vi "Read Target-FIFO 16ch.vi"(9 "ready for input":bool, 11 "channel number":u8) -> (4 "16xIQData":T1(array[cluster]) {"I" format="%.18g"; "Q" format="%.18g"}, 10 "Output Valid":bool)   [LabVIEW 2015, in "DDC_7976R_v1.lvlib"]
uses:
  DDC_7976R_v1.lvlib
types:
  T1 = cluster{"I":fxp<+/-,18,1>, "Q":fxp<+/-,18,1>, "overflow":bool}[]
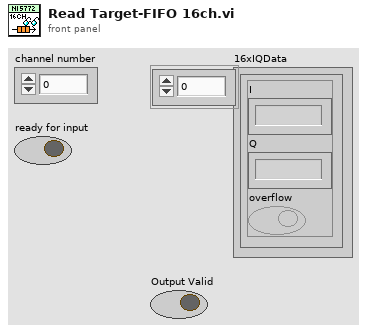
[diagram p1: front panel]
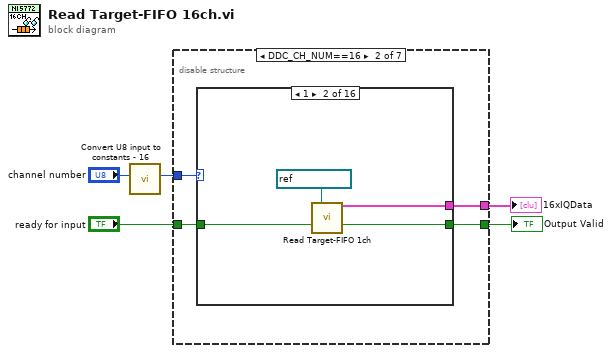
[diagram p0: block diagram]
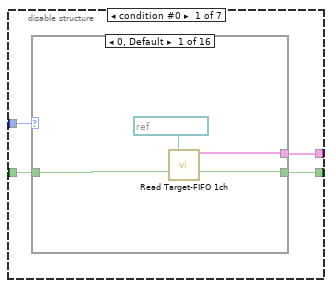
[diagram p2: hidden frame]
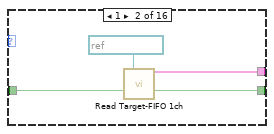
[diagram p3: hidden frame]
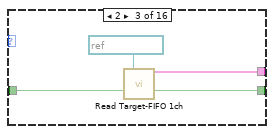
[diagram p4: hidden frame]
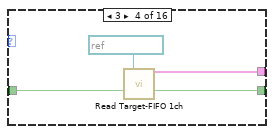
[diagram p5: hidden frame]
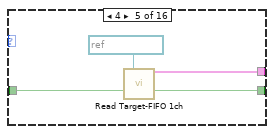
[diagram p6: hidden frame]
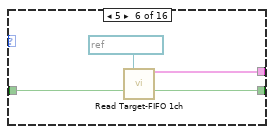
[diagram p7: hidden frame]
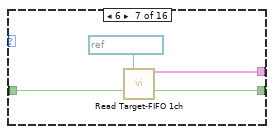
[diagram p8: hidden frame]
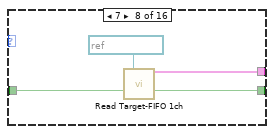
[diagram p9: hidden frame]
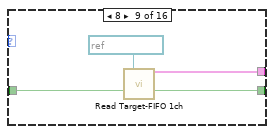
[diagram p10: hidden frame]
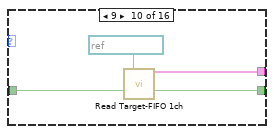
[diagram p11: hidden frame]
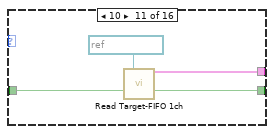
[diagram p12: hidden frame]
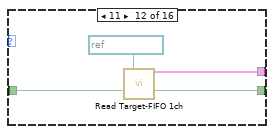
[diagram p13: hidden frame]
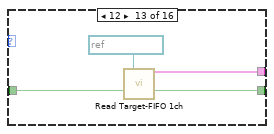
[diagram p14: hidden frame]
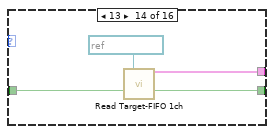
[diagram p15: hidden frame]
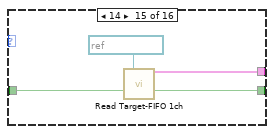
[diagram p16: hidden frame]
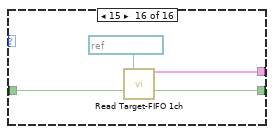
[diagram p17: hidden frame]
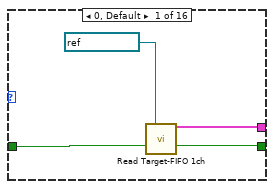
[diagram p18: hidden frame]
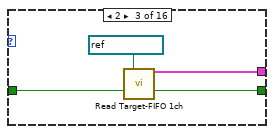
[diagram p19: hidden frame]
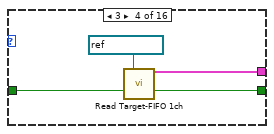
[diagram p20: hidden frame]
diagram:
  n1 = call "Convert U8 input to constants - 16.vi"("input U8"="channel number") -> ("output U8"=w1:u8)  [unwired: 10 in]
  n2 = disable-structure shown="DDC_CH_NUM==16" {
    disable-tunnel: [w9 w77 w145 w213 w281 w349 w415] -> w5
    disable-tunnel: [w8 w76 w144 w212 w280 w348 w416] -> w4
    disable-tunnel: "ready for input" -> [w7 w75 w143 w211 w279 w347 w414]
    disable-tunnel: w1 -> [w6 w74 w142 w210 w278 w346 _]
    frame condition #0 {
      n3 = case shown="0, Default" w6 {
        tunnel: w7 -> [w12 w16 w20 w24 w28 w32 w36 w40 w44 w48 w52 w56 w60 w64 w68 w72]
        tunnel: [w10 w15 w19 w23 w27 w31 w35 w39 w43 w47 w51 w55 w59 w63 w67 w71] -> w8
        tunnel: [w11 w14 w18 w22 w26 w30 w34 w38 w42 w46 w50 w54 w58 w62 w66 w70] -> w9
        frame 0, Default {
          n4 = call "Read Target-FIFO 1ch.vi"("FIFO In"=refnum<k21> "FIFO-000", "ready for input"=w12) -> ("16xIQData"=w10:T1, "Output Valid"=w11:bool)  [unwired: 12 in]
        }
        frame 1 {
          n5 = call "Read Target-FIFO 1ch.vi"("FIFO In"=refnum<k21> "FIFO-001", "ready for input"=w16) -> ("16xIQData"=w15:T1, "Output Valid"=w14:bool)  [unwired: 12 in]
        }
        frame 2 {
          n6 = call "Read Target-FIFO 1ch.vi"("FIFO In"=refnum<k21> "FIFO-002", "ready for input"=w20) -> ("16xIQData"=w19:T1, "Output Valid"=w18:bool)  [unwired: 12 in]
        }
        frame 3 {
          n7 = call "Read Target-FIFO 1ch.vi"("FIFO In"=refnum<k21> "FIFO-003", "ready for input"=w24) -> ("16xIQData"=w23:T1, "Output Valid"=w22:bool)  [unwired: 12 in]
        }
        frame 4 {
          n8 = call "Read Target-FIFO 1ch.vi"("FIFO In"=refnum<k21> "FIFO-004", "ready for input"=w28) -> ("16xIQData"=w27:T1, "Output Valid"=w26:bool)  [unwired: 12 in]
        }
        frame 5 {
          n9 = call "Read Target-FIFO 1ch.vi"("FIFO In"=refnum<k21> "FIFO-005", "ready for input"=w32) -> ("16xIQData"=w31:T1, "Output Valid"=w30:bool)  [unwired: 12 in]
        }
        frame 6 {
          n10 = call "Read Target-FIFO 1ch.vi"("FIFO In"=refnum<k21> "FIFO-006", "ready for input"=w36) -> ("16xIQData"=w35:T1, "Output Valid"=w34:bool)  [unwired: 12 in]
        }
        frame 7 {
          n11 = call "Read Target-FIFO 1ch.vi"("FIFO In"=refnum<k21> "FIFO-007", "ready for input"=w40) -> ("16xIQData"=w39:T1, "Output Valid"=w38:bool)  [unwired: 12 in]
        }
        frame 8 {
          n12 = call "Read Target-FIFO 1ch.vi"("FIFO In"=refnum<k21> "FIFO-008", "ready for input"=w44) -> ("16xIQData"=w43:T1, "Output Valid"=w42:bool)  [unwired: 12 in]
        }
        frame 9 {
          n13 = call "Read Target-FIFO 1ch.vi"("FIFO In"=refnum<k21> "FIFO-009", "ready for input"=w48) -> ("16xIQData"=w47:T1, "Output Valid"=w46:bool)  [unwired: 12 in]
        }
        frame 10 {
          n14 = call "Read Target-FIFO 1ch.vi"("FIFO In"=refnum<k21> "FIFO-010", "ready for input"=w52) -> ("16xIQData"=w51:T1, "Output Valid"=w50:bool)  [unwired: 12 in]
        }
        frame 11 {
          n15 = call "Read Target-FIFO 1ch.vi"("FIFO In"=refnum<k21> "FIFO-011", "ready for input"=w56) -> ("16xIQData"=w55:T1, "Output Valid"=w54:bool)  [unwired: 12 in]
        }
        frame 12 {
          n16 = call "Read Target-FIFO 1ch.vi"("FIFO In"=refnum<k21> "FIFO-012", "ready for input"=w60) -> ("16xIQData"=w59:T1, "Output Valid"=w58:bool)  [unwired: 12 in]
        }
        frame 13 {
          n17 = call "Read Target-FIFO 1ch.vi"("FIFO In"=refnum<k21> "FIFO-013", "ready for input"=w64) -> ("16xIQData"=w63:T1, "Output Valid"=w62:bool)  [unwired: 12 in]
        }
        frame 14 {
          n18 = call "Read Target-FIFO 1ch.vi"("FIFO In"=refnum<k21> "FIFO-014", "ready for input"=w68) -> ("16xIQData"=w67:T1, "Output Valid"=w66:bool)  [unwired: 12 in]
        }
        frame 15 {
          n19 = call "Read Target-FIFO 1ch.vi"("FIFO In"=refnum<k21> "FIFO-015", "ready for input"=w72) -> ("16xIQData"=w71:T1, "Output Valid"=w70:bool)  [unwired: 12 in]
        }
      }
    }
    frame condition #1 (active) {
      n20 = case shown="1" w74 {
        tunnel: w75 -> [w80 w84 w88 w92 w96 w100 w104 w108 w112 w116 w120 w124 w128 w132 w136 w140]
        tunnel: [w78 w83 w87 w91 w95 w99 w103 w107 w111 w115 w119 w123 w127 w131 w135 w139] -> w76
        tunnel: [w79 w82 w86 w90 w94 w98 w102 w106 w110 w114 w118 w122 w126 w130 w134 w138] -> w77
        frame 0, Default {
          n21 = call "Read Target-FIFO 1ch.vi"("FIFO In"=refnum<k21> "FIFO-000", "ready for input"=w80) -> ("16xIQData"=w78:T1, "Output Valid"=w79:bool)  [unwired: 12 in]
        }
        frame 1 {
          n22 = call "Read Target-FIFO 1ch.vi"("FIFO In"=refnum<k21> "FIFO-001", "ready for input"=w84) -> ("16xIQData"=w83:T1, "Output Valid"=w82:bool)  [unwired: 12 in]
        }
        frame 2 {
          n23 = call "Read Target-FIFO 1ch.vi"("FIFO In"=refnum<k21> "FIFO-002", "ready for input"=w88) -> ("16xIQData"=w87:T1, "Output Valid"=w86:bool)  [unwired: 12 in]
        }
        frame 3 {
          n24 = call "Read Target-FIFO 1ch.vi"("FIFO In"=refnum<k21> "FIFO-003", "ready for input"=w92) -> ("16xIQData"=w91:T1, "Output Valid"=w90:bool)  [unwired: 12 in]
        }
        frame 4 {
          n25 = call "Read Target-FIFO 1ch.vi"("FIFO In"=refnum<k21> "FIFO-004", "ready for input"=w96) -> ("16xIQData"=w95:T1, "Output Valid"=w94:bool)  [unwired: 12 in]
        }
        frame 5 {
          n26 = call "Read Target-FIFO 1ch.vi"("FIFO In"=refnum<k21> "FIFO-005", "ready for input"=w100) -> ("16xIQData"=w99:T1, "Output Valid"=w98:bool)  [unwired: 12 in]
        }
        frame 6 {
          n27 = call "Read Target-FIFO 1ch.vi"("FIFO In"=refnum<k21> "FIFO-006", "ready for input"=w104) -> ("16xIQData"=w103:T1, "Output Valid"=w102:bool)  [unwired: 12 in]
        }
        frame 7 {
          n28 = call "Read Target-FIFO 1ch.vi"("FIFO In"=refnum<k21> "FIFO-007", "ready for input"=w108) -> ("16xIQData"=w107:T1, "Output Valid"=w106:bool)  [unwired: 12 in]
        }
        frame 8 {
          n29 = call "Read Target-FIFO 1ch.vi"("FIFO In"=refnum<k21> "FIFO-008", "ready for input"=w112) -> ("16xIQData"=w111:T1, "Output Valid"=w110:bool)  [unwired: 12 in]
        }
        frame 9 {
          n30 = call "Read Target-FIFO 1ch.vi"("FIFO In"=refnum<k21> "FIFO-009", "ready for input"=w116) -> ("16xIQData"=w115:T1, "Output Valid"=w114:bool)  [unwired: 12 in]
        }
        frame 10 {
          n31 = call "Read Target-FIFO 1ch.vi"("FIFO In"=refnum<k21> "FIFO-010", "ready for input"=w120) -> ("16xIQData"=w119:T1, "Output Valid"=w118:bool)  [unwired: 12 in]
        }
        frame 11 {
          n32 = call "Read Target-FIFO 1ch.vi"("FIFO In"=refnum<k21> "FIFO-011", "ready for input"=w124) -> ("16xIQData"=w123:T1, "Output Valid"=w122:bool)  [unwired: 12 in]
        }
        frame 12 {
          n33 = call "Read Target-FIFO 1ch.vi"("FIFO In"=refnum<k21> "FIFO-012", "ready for input"=w128) -> ("16xIQData"=w127:T1, "Output Valid"=w126:bool)  [unwired: 12 in]
        }
        frame 13 {
          n34 = call "Read Target-FIFO 1ch.vi"("FIFO In"=refnum<k21> "FIFO-013", "ready for input"=w132) -> ("16xIQData"=w131:T1, "Output Valid"=w130:bool)  [unwired: 12 in]
        }
        frame 14 {
          n35 = call "Read Target-FIFO 1ch.vi"("FIFO In"=refnum<k21> "FIFO-014", "ready for input"=w136) -> ("16xIQData"=w135:T1, "Output Valid"=w134:bool)  [unwired: 12 in]
        }
        frame 15 {
          n36 = call "Read Target-FIFO 1ch.vi"("FIFO In"=refnum<k21> "FIFO-015", "ready for input"=w140) -> ("16xIQData"=w139:T1, "Output Valid"=w138:bool)  [unwired: 12 in]
        }
      }
    }
    frame condition #2 {
      n37 = case shown="0, Default" w142 {
        tunnel: w143 -> [w148 w152 w156 w160 w164 w168 w172 w176 w180 w184 w188 w192 w196 w200 w204 w208]
        tunnel: [w146 w151 w155 w159 w163 w167 w171 w175 w179 w183 w187 w191 w195 w199 w203 w207] -> w144
        tunnel: [w147 w150 w154 w158 w162 w166 w170 w174 w178 w182 w186 w190 w194 w198 w202 w206] -> w145
        frame 0, Default {
          n38 = call "Read Target-FIFO 1ch.vi"("FIFO In"=refnum<k21> "FIFO-000", "ready for input"=w148) -> ("16xIQData"=w146:T1, "Output Valid"=w147:bool)  [unwired: 12 in]
        }
        frame 1 {
          n39 = call "Read Target-FIFO 1ch.vi"("FIFO In"=refnum<k21> "FIFO-001", "ready for input"=w152) -> ("16xIQData"=w151:T1, "Output Valid"=w150:bool)  [unwired: 12 in]
        }
        frame 2 {
          n40 = call "Read Target-FIFO 1ch.vi"("FIFO In"=refnum<k21> "FIFO-002", "ready for input"=w156) -> ("16xIQData"=w155:T1, "Output Valid"=w154:bool)  [unwired: 12 in]
        }
        frame 3 {
          n41 = call "Read Target-FIFO 1ch.vi"("FIFO In"=refnum<k21> "FIFO-003", "ready for input"=w160) -> ("16xIQData"=w159:T1, "Output Valid"=w158:bool)  [unwired: 12 in]
        }
        frame 4 {
          n42 = call "Read Target-FIFO 1ch.vi"("FIFO In"=refnum<k21> "FIFO-004", "ready for input"=w164) -> ("16xIQData"=w163:T1, "Output Valid"=w162:bool)  [unwired: 12 in]
        }
        frame 5 {
          n43 = call "Read Target-FIFO 1ch.vi"("FIFO In"=refnum<k21> "FIFO-005", "ready for input"=w168) -> ("16xIQData"=w167:T1, "Output Valid"=w166:bool)  [unwired: 12 in]
        }
        frame 6 {
          n44 = call "Read Target-FIFO 1ch.vi"("FIFO In"=refnum<k21> "FIFO-006", "ready for input"=w172) -> ("16xIQData"=w171:T1, "Output Valid"=w170:bool)  [unwired: 12 in]
        }
        frame 7 {
          n45 = call "Read Target-FIFO 1ch.vi"("FIFO In"=refnum<k21> "FIFO-007", "ready for input"=w176) -> ("16xIQData"=w175:T1, "Output Valid"=w174:bool)  [unwired: 12 in]
        }
        frame 8 {
          n46 = call "Read Target-FIFO 1ch.vi"("FIFO In"=refnum<k21> "FIFO-008", "ready for input"=w180) -> ("16xIQData"=w179:T1, "Output Valid"=w178:bool)  [unwired: 12 in]
        }
        frame 9 {
          n47 = call "Read Target-FIFO 1ch.vi"("FIFO In"=refnum<k21> "FIFO-009", "ready for input"=w184) -> ("16xIQData"=w183:T1, "Output Valid"=w182:bool)  [unwired: 12 in]
        }
        frame 10 {
          n48 = call "Read Target-FIFO 1ch.vi"("FIFO In"=refnum<k21> "FIFO-010", "ready for input"=w188) -> ("16xIQData"=w187:T1, "Output Valid"=w186:bool)  [unwired: 12 in]
        }
        frame 11 {
          n49 = call "Read Target-FIFO 1ch.vi"("FIFO In"=refnum<k21> "FIFO-011", "ready for input"=w192) -> ("16xIQData"=w191:T1, "Output Valid"=w190:bool)  [unwired: 12 in]
        }
        frame 12 {
          n50 = call "Read Target-FIFO 1ch.vi"("FIFO In"=refnum<k21> "FIFO-012", "ready for input"=w196) -> ("16xIQData"=w195:T1, "Output Valid"=w194:bool)  [unwired: 12 in]
        }
        frame 13 {
          n51 = call "Read Target-FIFO 1ch.vi"("FIFO In"=refnum<k21> "FIFO-013", "ready for input"=w200) -> ("16xIQData"=w199:T1, "Output Valid"=w198:bool)  [unwired: 12 in]
        }
        frame 14 {
          n52 = call "Read Target-FIFO 1ch.vi"("FIFO In"=refnum<k21> "FIFO-014", "ready for input"=w204) -> ("16xIQData"=w203:T1, "Output Valid"=w202:bool)  [unwired: 12 in]
        }
        frame 15 {
          n53 = call "Read Target-FIFO 1ch.vi"("FIFO In"=refnum<k21> "FIFO-015", "ready for input"=w208) -> ("16xIQData"=w207:T1, "Output Valid"=w206:bool)  [unwired: 12 in]
        }
      }
    }
    frame condition #3 {
      n54 = case shown="0, Default" w210 {
        tunnel: w211 -> [w216 w220 w224 w228 w232 w236 w240 w244 w248 w252 w256 w260 w264 w268 w272 w276]
        tunnel: [w214 w219 w223 w227 w231 w235 w239 w243 w247 w251 w255 w259 w263 w267 w271 w275] -> w212
        tunnel: [w215 w218 w222 w226 w230 w234 w238 w242 w246 w250 w254 w258 w262 w266 w270 w274] -> w213
        frame 0, Default {
          n55 = call "Read Target-FIFO 1ch.vi"("FIFO In"=refnum<k21> "FIFO-000", "ready for input"=w216) -> ("16xIQData"=w214:T1, "Output Valid"=w215:bool)  [unwired: 12 in]
        }
        frame 1 {
          n56 = call "Read Target-FIFO 1ch.vi"("FIFO In"=refnum<k21> "FIFO-001", "ready for input"=w220) -> ("16xIQData"=w219:T1, "Output Valid"=w218:bool)  [unwired: 12 in]
        }
        frame 2 {
          n57 = call "Read Target-FIFO 1ch.vi"("FIFO In"=refnum<k21> "FIFO-002", "ready for input"=w224) -> ("16xIQData"=w223:T1, "Output Valid"=w222:bool)  [unwired: 12 in]
        }
        frame 3 {
          n58 = call "Read Target-FIFO 1ch.vi"("FIFO In"=refnum<k21> "FIFO-003", "ready for input"=w228) -> ("16xIQData"=w227:T1, "Output Valid"=w226:bool)  [unwired: 12 in]
        }
        frame 4 {
          n59 = call "Read Target-FIFO 1ch.vi"("FIFO In"=refnum<k21> "FIFO-004", "ready for input"=w232) -> ("16xIQData"=w231:T1, "Output Valid"=w230:bool)  [unwired: 12 in]
        }
        frame 5 {
          n60 = call "Read Target-FIFO 1ch.vi"("FIFO In"=refnum<k21> "FIFO-005", "ready for input"=w236) -> ("16xIQData"=w235:T1, "Output Valid"=w234:bool)  [unwired: 12 in]
        }
        frame 6 {
          n61 = call "Read Target-FIFO 1ch.vi"("FIFO In"=refnum<k21> "FIFO-006", "ready for input"=w240) -> ("16xIQData"=w239:T1, "Output Valid"=w238:bool)  [unwired: 12 in]
        }
        frame 7 {
          n62 = call "Read Target-FIFO 1ch.vi"("FIFO In"=refnum<k21> "FIFO-007", "ready for input"=w244) -> ("16xIQData"=w243:T1, "Output Valid"=w242:bool)  [unwired: 12 in]
        }
        frame 8 {
          n63 = call "Read Target-FIFO 1ch.vi"("FIFO In"=refnum<k21> "FIFO-008", "ready for input"=w248) -> ("16xIQData"=w247:T1, "Output Valid"=w246:bool)  [unwired: 12 in]
        }
        frame 9 {
          n64 = call "Read Target-FIFO 1ch.vi"("FIFO In"=refnum<k21> "FIFO-009", "ready for input"=w252) -> ("16xIQData"=w251:T1, "Output Valid"=w250:bool)  [unwired: 12 in]
        }
        frame 10 {
          n65 = call "Read Target-FIFO 1ch.vi"("FIFO In"=refnum<k21> "FIFO-010", "ready for input"=w256) -> ("16xIQData"=w255:T1, "Output Valid"=w254:bool)  [unwired: 12 in]
        }
        frame 11 {
          n66 = call "Read Target-FIFO 1ch.vi"("FIFO In"=refnum<k21> "FIFO-011", "ready for input"=w260) -> ("16xIQData"=w259:T1, "Output Valid"=w258:bool)  [unwired: 12 in]
        }
        frame 12 {
          n67 = call "Read Target-FIFO 1ch.vi"("FIFO In"=refnum<k21> "FIFO-012", "ready for input"=w264) -> ("16xIQData"=w263:T1, "Output Valid"=w262:bool)  [unwired: 12 in]
        }
        frame 13 {
          n68 = call "Read Target-FIFO 1ch.vi"("FIFO In"=refnum<k21> "FIFO-013", "ready for input"=w268) -> ("16xIQData"=w267:T1, "Output Valid"=w266:bool)  [unwired: 12 in]
        }
        frame 14 {
          n69 = call "Read Target-FIFO 1ch.vi"("FIFO In"=refnum<k21> "FIFO-014", "ready for input"=w272) -> ("16xIQData"=w271:T1, "Output Valid"=w270:bool)  [unwired: 12 in]
        }
        frame 15 {
          n70 = call "Read Target-FIFO 1ch.vi"("FIFO In"=refnum<k21> "FIFO-015", "ready for input"=w276) -> ("16xIQData"=w275:T1, "Output Valid"=w274:bool)  [unwired: 12 in]
        }
      }
    }
    frame condition #4 {
      n71 = case shown="0, Default" w278 {
        tunnel: w279 -> [w284 w288 w292 w296 w300 w304 w308 w312 w316 w320 w324 w328 w332 w336 w340 w344]
        tunnel: [w282 w287 w291 w295 w299 w303 w307 w311 w315 w319 w323 w327 w331 w335 w339 w343] -> w280
        tunnel: [w283 w286 w290 w294 w298 w302 w306 w310 w314 w318 w322 w326 w330 w334 w338 w342] -> w281
        frame 0, Default {
          n72 = call "Read Target-FIFO 1ch.vi"("FIFO In"=refnum<k21> "FIFO-000", "ready for input"=w284) -> ("16xIQData"=w282:T1, "Output Valid"=w283:bool)  [unwired: 12 in]
        }
        frame 1 {
          n73 = call "Read Target-FIFO 1ch.vi"("FIFO In"=refnum<k21> "FIFO-001", "ready for input"=w288) -> ("16xIQData"=w287:T1, "Output Valid"=w286:bool)  [unwired: 12 in]
        }
        frame 2 {
          n74 = call "Read Target-FIFO 1ch.vi"("FIFO In"=refnum<k21> "FIFO-002", "ready for input"=w292) -> ("16xIQData"=w291:T1, "Output Valid"=w290:bool)  [unwired: 12 in]
        }
        frame 3 {
          n75 = call "Read Target-FIFO 1ch.vi"("FIFO In"=refnum<k21> "FIFO-003", "ready for input"=w296) -> ("16xIQData"=w295:T1, "Output Valid"=w294:bool)  [unwired: 12 in]
        }
        frame 4 {
          n76 = call "Read Target-FIFO 1ch.vi"("FIFO In"=refnum<k21> "FIFO-004", "ready for input"=w300) -> ("16xIQData"=w299:T1, "Output Valid"=w298:bool)  [unwired: 12 in]
        }
        frame 5 {
          n77 = call "Read Target-FIFO 1ch.vi"("FIFO In"=refnum<k21> "FIFO-005", "ready for input"=w304) -> ("16xIQData"=w303:T1, "Output Valid"=w302:bool)  [unwired: 12 in]
        }
        frame 6 {
          n78 = call "Read Target-FIFO 1ch.vi"("FIFO In"=refnum<k21> "FIFO-006", "ready for input"=w308) -> ("16xIQData"=w307:T1, "Output Valid"=w306:bool)  [unwired: 12 in]
        }
        frame 7 {
          n79 = call "Read Target-FIFO 1ch.vi"("FIFO In"=refnum<k21> "FIFO-007", "ready for input"=w312) -> ("16xIQData"=w311:T1, "Output Valid"=w310:bool)  [unwired: 12 in]
        }
        frame 8 {
          n80 = call "Read Target-FIFO 1ch.vi"("FIFO In"=refnum<k21> "FIFO-008", "ready for input"=w316) -> ("16xIQData"=w315:T1, "Output Valid"=w314:bool)  [unwired: 12 in]
        }
        frame 9 {
          n81 = call "Read Target-FIFO 1ch.vi"("FIFO In"=refnum<k21> "FIFO-009", "ready for input"=w320) -> ("16xIQData"=w319:T1, "Output Valid"=w318:bool)  [unwired: 12 in]
        }
        frame 10 {
          n82 = call "Read Target-FIFO 1ch.vi"("FIFO In"=refnum<k21> "FIFO-010", "ready for input"=w324) -> ("16xIQData"=w323:T1, "Output Valid"=w322:bool)  [unwired: 12 in]
        }
        frame 11 {
          n83 = call "Read Target-FIFO 1ch.vi"("FIFO In"=refnum<k21> "FIFO-011", "ready for input"=w328) -> ("16xIQData"=w327:T1, "Output Valid"=w326:bool)  [unwired: 12 in]
        }
        frame 12 {
          n84 = call "Read Target-FIFO 1ch.vi"("FIFO In"=refnum<k21> "FIFO-012", "ready for input"=w332) -> ("16xIQData"=w331:T1, "Output Valid"=w330:bool)  [unwired: 12 in]
        }
        frame 13 {
          n85 = call "Read Target-FIFO 1ch.vi"("FIFO In"=refnum<k21> "FIFO-013", "ready for input"=w336) -> ("16xIQData"=w335:T1, "Output Valid"=w334:bool)  [unwired: 12 in]
        }
        frame 14 {
          n86 = call "Read Target-FIFO 1ch.vi"("FIFO In"=refnum<k21> "FIFO-014", "ready for input"=w340) -> ("16xIQData"=w339:T1, "Output Valid"=w338:bool)  [unwired: 12 in]
        }
        frame 15 {
          n87 = call "Read Target-FIFO 1ch.vi"("FIFO In"=refnum<k21> "FIFO-015", "ready for input"=w344) -> ("16xIQData"=w343:T1, "Output Valid"=w342:bool)  [unwired: 12 in]
        }
      }
    }
    frame condition #5 {
      n88 = case shown="0, Default" w346 {
        tunnel: w347 -> [w352 w356 w360 w364 w368 w372 w376 w380 w384 w388 w392 w396 w400 w404 w408 w412]
        tunnel: [w350 w355 w359 w363 w367 w371 w375 w379 w383 w387 w391 w395 w399 w403 w407 w411] -> w348
        tunnel: [w351 w354 w358 w362 w366 w370 w374 w378 w382 w386 w390 w394 w398 w402 w406 w410] -> w349
        frame 0, Default {
          n89 = call "Read Target-FIFO 1ch.vi"("FIFO In"=refnum<k21> "FIFO-000", "ready for input"=w352) -> ("16xIQData"=w350:T1, "Output Valid"=w351:bool)  [unwired: 12 in]
        }
        frame 1 {
          n90 = call "Read Target-FIFO 1ch.vi"("FIFO In"=refnum<k21> "FIFO-001", "ready for input"=w356) -> ("16xIQData"=w355:T1, "Output Valid"=w354:bool)  [unwired: 12 in]
        }
        frame 2 {
          n91 = call "Read Target-FIFO 1ch.vi"("FIFO In"=refnum<k21> "FIFO-002", "ready for input"=w360) -> ("16xIQData"=w359:T1, "Output Valid"=w358:bool)  [unwired: 12 in]
        }
        frame 3 {
          n92 = call "Read Target-FIFO 1ch.vi"("FIFO In"=refnum<k21> "FIFO-003", "ready for input"=w364) -> ("16xIQData"=w363:T1, "Output Valid"=w362:bool)  [unwired: 12 in]
        }
        frame 4 {
          n93 = call "Read Target-FIFO 1ch.vi"("FIFO In"=refnum<k21> "FIFO-004", "ready for input"=w368) -> ("16xIQData"=w367:T1, "Output Valid"=w366:bool)  [unwired: 12 in]
        }
        frame 5 {
          n94 = call "Read Target-FIFO 1ch.vi"("FIFO In"=refnum<k21> "FIFO-005", "ready for input"=w372) -> ("16xIQData"=w371:T1, "Output Valid"=w370:bool)  [unwired: 12 in]
        }
        frame 6 {
          n95 = call "Read Target-FIFO 1ch.vi"("FIFO In"=refnum<k21> "FIFO-006", "ready for input"=w376) -> ("16xIQData"=w375:T1, "Output Valid"=w374:bool)  [unwired: 12 in]
        }
        frame 7 {
          n96 = call "Read Target-FIFO 1ch.vi"("FIFO In"=refnum<k21> "FIFO-007", "ready for input"=w380) -> ("16xIQData"=w379:T1, "Output Valid"=w378:bool)  [unwired: 12 in]
        }
        frame 8 {
          n97 = call "Read Target-FIFO 1ch.vi"("FIFO In"=refnum<k21> "FIFO-008", "ready for input"=w384) -> ("16xIQData"=w383:T1, "Output Valid"=w382:bool)  [unwired: 12 in]
        }
        frame 9 {
          n98 = call "Read Target-FIFO 1ch.vi"("FIFO In"=refnum<k21> "FIFO-009", "ready for input"=w388) -> ("16xIQData"=w387:T1, "Output Valid"=w386:bool)  [unwired: 12 in]
        }
        frame 10 {
          n99 = call "Read Target-FIFO 1ch.vi"("FIFO In"=refnum<k21> "FIFO-010", "ready for input"=w392) -> ("16xIQData"=w391:T1, "Output Valid"=w390:bool)  [unwired: 12 in]
        }
        frame 11 {
          n100 = call "Read Target-FIFO 1ch.vi"("FIFO In"=refnum<k21> "FIFO-011", "ready for input"=w396) -> ("16xIQData"=w395:T1, "Output Valid"=w394:bool)  [unwired: 12 in]
        }
        frame 12 {
          n101 = call "Read Target-FIFO 1ch.vi"("FIFO In"=refnum<k21> "FIFO-012", "ready for input"=w400) -> ("16xIQData"=w399:T1, "Output Valid"=w398:bool)  [unwired: 12 in]
        }
        frame 13 {
          n102 = call "Read Target-FIFO 1ch.vi"("FIFO In"=refnum<k21> "FIFO-013", "ready for input"=w404) -> ("16xIQData"=w403:T1, "Output Valid"=w402:bool)  [unwired: 12 in]
        }
        frame 14 {
          n103 = call "Read Target-FIFO 1ch.vi"("FIFO In"=refnum<k21> "FIFO-014", "ready for input"=w408) -> ("16xIQData"=w407:T1, "Output Valid"=w406:bool)  [unwired: 12 in]
        }
        frame 15 {
          n104 = call "Read Target-FIFO 1ch.vi"("FIFO In"=refnum<k21> "FIFO-015", "ready for input"=w412) -> ("16xIQData"=w411:T1, "Output Valid"=w410:bool)  [unwired: 12 in]
        }
      }
    }
    frame condition #6 {
      n105 = call "Read Target-FIFO 1ch.vi"("FIFO In"=refnum<k21> "FIFO-000", "ready for input"=w414) -> ("16xIQData"=w416:T1, "Output Valid"=w415:bool)  [unwired: 12 in]
    }
  }
  "Output Valid" <- w5
  "16xIQData" <- w4
